vi "Get Tests Events by Key.vi"(8 "error in (no error)":errorcluster, 10 "Key (Test ID)":string, 11 "Test Event Storage in":refnum<class "Test Event Storage.lvclass">) -> (0 "error out":errorcluster, 1 "Assertions":T1[](array[typedef]), 3 "Test Event Storage out":refnum<class "Test Event Storage.lvclass">)   [LabVIEW 2013, in "Caraya.lvlib" / "Test Event Storage.lvclass"]
uses:
  Test Event Storage.lvclass
  Test Result/Assert Event Data.ctl
  Test Event Storage.lvclass/Test Event Storage.ctl
  test store -- cluster.ctl
  Test Manager Message Test/TestManagerMsg.Test.lvclass
  assert store -- cluster.ctl
  Test Manager Message Assertion/TestManagerMsg.Assertion.lvclass
  Test Manager Message Verbose/TestManagerMsg.Verbose.lvclass
  Test Result/Test Result.lvclass
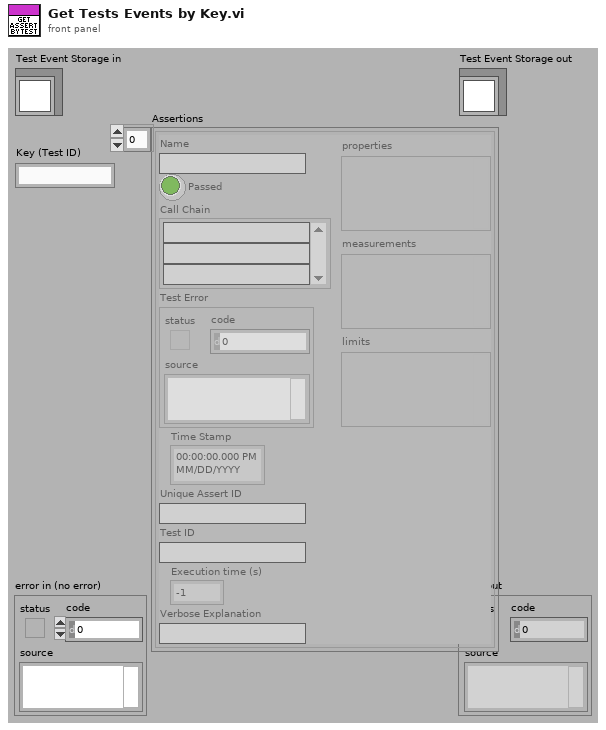
[diagram p1: front panel]
types:
  T1 = typedef "Caraya.lvlib/Test Result.lvclass/Assert Event Data.ctl" = cluster{"Name":string, "Passed":bool, "Call Chain":string[], "Test Error":errorcluster, "Time Stamp":timestamp, "Unique Assert ID":string, "Test ID":string, "Execution time (s)":dbl, "Verbose Explanation":string, "properties":variant, "measurements":variant, "limits":variant}
  T2 = typedef "Caraya.lvlib/Test Event Storage.lvclass/assert store -- cluster.ctl" = cluster{"Assertion":refnum<class "TestManagerMsg.Assertion.lvclass">, "Explanation":refnum<class "TestManagerMsg.Verbose.lvclass">, "properties":variant, "measurements":variant, "limits":variant}
  T3 = typedef "Caraya.lvlib/Test Event Storage.lvclass/test store -- cluster.ctl" = cluster{"Test":refnum<class "TestManagerMsg.Test.lvclass">, "Defined":bool, "Passed":bool, "properties":variant, "assert-ids":variant}
  T4 = typedef "Caraya.lvlib/Test Event Storage.lvclass/store version -- enum.ctl" = enum16{"v1", "v2"}
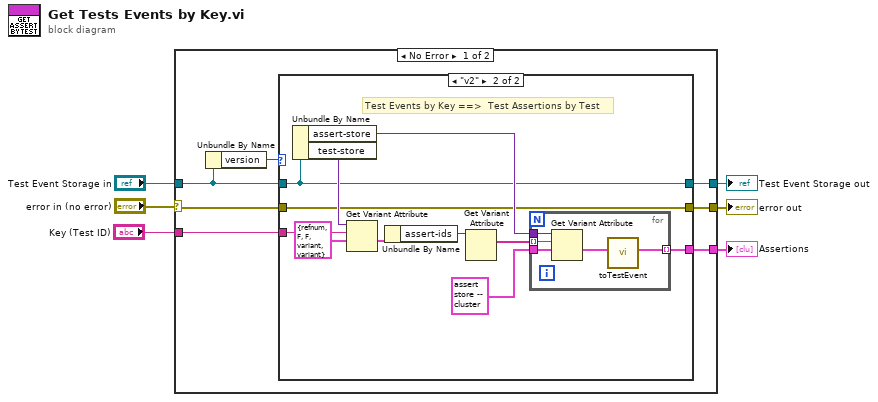
[diagram p0: block diagram]
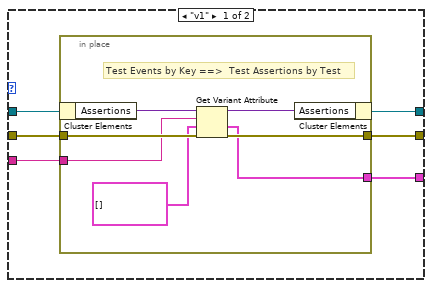
[diagram p2: hidden frame]
diagram:
  n1 = case shown="No Error" "error in (no error)" {
    selector: "error in (no error)" -> [w10 w44]
    tunnel: [w13 w44] -> w5
    tunnel: [w12 w43] -> w3
    tunnel: "Test Event Storage in" -> [w8 w43]
    tunnel: "Key (Test ID)" -> [w11 _]
    tunnel: [w9 _] -> w1
    frame No Error {
      n2 = Unbundle By Name(w8) -> ("version"=w7:T4)
      n3 = case shown="\"v2\"" w7 {
        tunnel: [w19 w31] -> w13
        tunnel: [w18 w32] -> w12
        tunnel: w11 -> [w17 w36]
        tunnel: w10 -> [w16 w31]
        tunnel: [w15 w30] -> w9
        tunnel: w8 -> [w14 w32]
        frame "v1" {
          n4 = in-place {
            in-place-border: w16 -> [w25]
            in-place-border: [w23] -> w19
            in-place-border: w17 -> [w22]
            in-place-border: [w20] -> w15
            # "Test Events by Key ==>  Test Assertions by Test"
            n5 = in-place-cluster #1(w14) -> ("Assertions"=w26:variant)
            n6 = Get Variant Attribute(Variant=w26, name=w22, default value (empty Variant)=T1[] [], error in=w25) -> (duplicate Variant=w24:variant, value=w20:T1[], error out=w23:errorcluster)  [unwired: 1 out]
            n7 = in-place-cluster #1("Assertions"=w24) -> (w18:refnum<class "Test Event Storage.lvclass">)
          }
        }
        frame "v2" {
          # "Test Events by Key ==>  Test Assertions by Test"
          n8 = Unbundle By Name(w32) -> ("assert-store"=w34:variant, "test-store"=w37:variant)
          n9 = Get Variant Attribute(Variant=w37, name=w36, default value (empty Variant)=T3 {"Test"=refnum, "Defined"=FALSE, "Passed"=FALSE, "properties"=variant, "assert-ids"=variant} ("test-store")) -> (value=w29:T3)  [unwired: 1 in, 3 out]
          n10 = Unbundle By Name(w29) -> ("assert-ids"=w28:variant)
          n11 = Get Variant Attribute(Variant=w28) -> (names=w27:string[])  [unwired: 3 in, 3 out]
          n12 = for {
            tunnel: w34 -> [w42]
            tunnel: w27 -> [w41] mode=indexing
            tunnel: T2 {"Assertion"=refnum, "Explanation"=refnum, "properties"=variant, "measurements"=variant, "limits"=variant} ("assert-store") -> [w40]
            tunnel: [w38] -> w30 mode=indexing
            n13 = Get Variant Attribute(Variant=w42, name=w41, default value (empty Variant)=w40) -> (value=w39:T2)  [unwired: 1 in, 3 out]
            n14 = call "toTestEvent.vi"("assert-store"=w39) -> ("Test Event"=w38:T1)  [unwired: 10 in]
          }
        }
      }
    }
    frame Error {
    }
  }
  "error out" <- w5
  "Test Event Storage out" <- w3
  "Assertions" <- w1
